vi "LSX Is Vel Single Axis.vi"(8 "error in (no error)":errorcluster, 9 "pdVel":dbl, 10 "lAxis":i32, 11 "lLSID":i32) -> (0 "error out":errorcluster, 1 "pdVel out":dbl, 3 "function return":i32)   [LabVIEW 2018, in "Tango.lvlib"]
doc: "TANGOAPI int TANGOCALL LSX_IsVelSingleAxis (int lLSID, int lAxis, double *pdVel);"
uses:
  <userlib>/Tango/Tango.lvlib
  <userlib>/Tango/Tango_DLL.dll
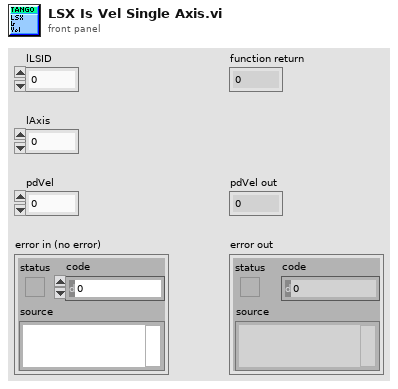
[diagram p1: front panel]
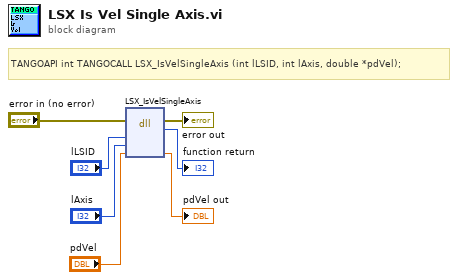
[diagram p0: block diagram]
diagram:
  # "TANGOAPI int TANGOCALL LSX_IsVelSingleAxis (int lLSID, int lAxis, double *pdVel);"
  n1 = dll-call lib="C:/Program Files (x86)/National Instruments/LabVIEW 2018/user.lib/Tango/Tango_DLL.*" fn="LSX_IsVelSingleAxis"(error in="error in (no error)", "lLSID"="lLSID", "lAxis"="lAxis", "pdVel"="pdVel") -> (error out=→"error out":errorcluster, →"function return":i32, "pdVel"=→"pdVel out":dbl)  [unwired: 4 in, 1 out]
